vi "humidity_sensing_v_2.vi"() -> ()   [LabVIEW 2014]
doc: "This example shows how to configure a measurement and take a reading."
uses:
  <instrlib>/Keithley 24XX/Public/Data/Read (Single Point).vi
  <instrlib>/Keithley 24XX/Keithley 24XX.lvlib
panel:
  in  "current multiplier":dbl=1000000.0
  out "Resistance Data":string
  in  "Resistance Data":path=path "C:/Users/Administrator/Documents/humidity_sensing_setup/data/dumb/data_dumb_1.txt"
  out "Current Data":string
  in  "Current Data":path=path "C:/Users/Administrator/Documents/humidity_sensing_setup/data/dumb/data_dumb.txt"
  in  "stop":bool
  in  "Sampling rate (ms/pt)":i32=1000
  out "Current Data Graph":sgl(graph)=0.0001831192
  out "Resistance Data Graph":sgl(graph)=5460.51
  in  "loop num":dbl=10000000000.0
  in  "Stop Voltage/Current":dbl=1.0
  in  "Step":dbl
  in  "Source Mode  (0: Voltage)":u16(ring) items=["Voltage", "Current"]
  in  "Compliance  Level (0.1)":dbl=1.0
  in  "Start Voltage/Current":dbl=1.0
  in  "Enable Resistance Auto Range (T:Enable)":bool
  in  "Enable Current Auto Range (T:Enable)":bool=TRUE
  in  "Enable Voltage Auto Range (T:Enable)":bool
  in  "Resistance Manual Range (1.0)":dbl=1.0
  in  "Current Manual Range (1.0)":dbl=1.0
  in  "Voltage Manual Range (1.0)":dbl=1.0
  out "Resistance":sgl
  out "Current":sgl
  out "Voltage":sgl
  in  "Serial Configuration":T1={"Baud Rate"=9600, "Parity"=0, "Data Bits"=8, "Stop Bits"=10, "Flow Control"=0} {"Flow Control" items=["None", "XON/XOFF", "RTS/CTS", "XON/XOFF & RTS/CTS", "DTR/DSR", "XON/XOFF & DTR/DSR"]; "Stop Bits" items=["1.0"=10, "1.5"=15, "2.0"=20]; "Data Bits" items=["7"=7, "8"=8]; "Parity" items=["None", "Odd", "Even", "Mark", "Space"]; "Baud Rate" items=["300"=300, "600"=600, "1200"=1200, "2400"=2400, "4800"=4800, "9600"=9600, "19200"=19200]}
  in  "VISA resource name":refnum<visa-resource-name>="GPIB9::24::INSTR"
  # "NanoBEEs 2016-Humidity Chamber Setup v2.0"
  # "Source Settings"
  # "GPIB9::24::INSTR"
  # "Voltage Range Settings"
  # "Current Range Settings"
  # "This multiplies the current value\nwith the number that entered, in order\nto  graph lower current values."
  # "Resistance Range Settings"
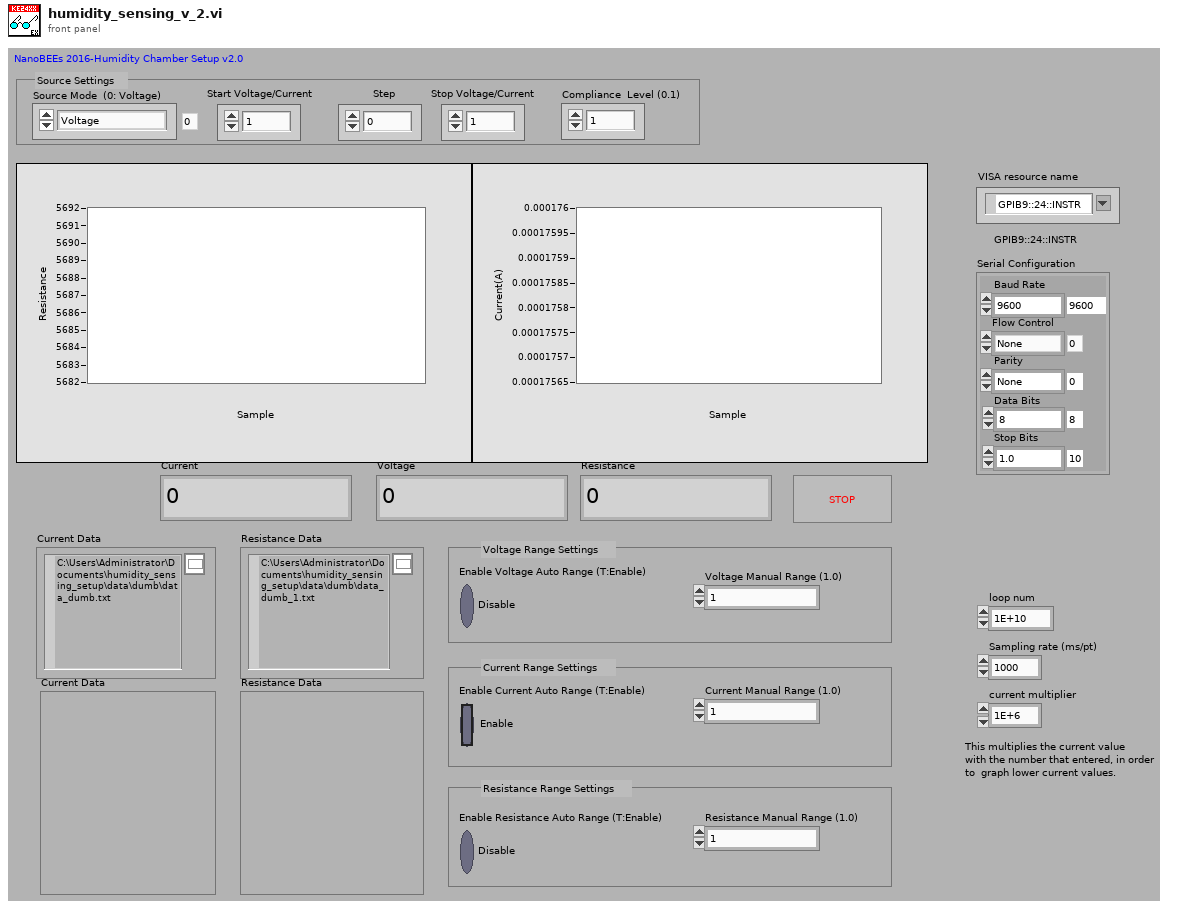
[diagram p1: front panel]
types:
  T1 = cluster{"Baud Rate":u32, "Parity":u16, "Data Bits":u16, "Stop Bits":u16, "Flow Control":u16}
  T2 = enum16{"open", "replace", "create", "open or create", "replace or create", "replace or create with confirmation"}
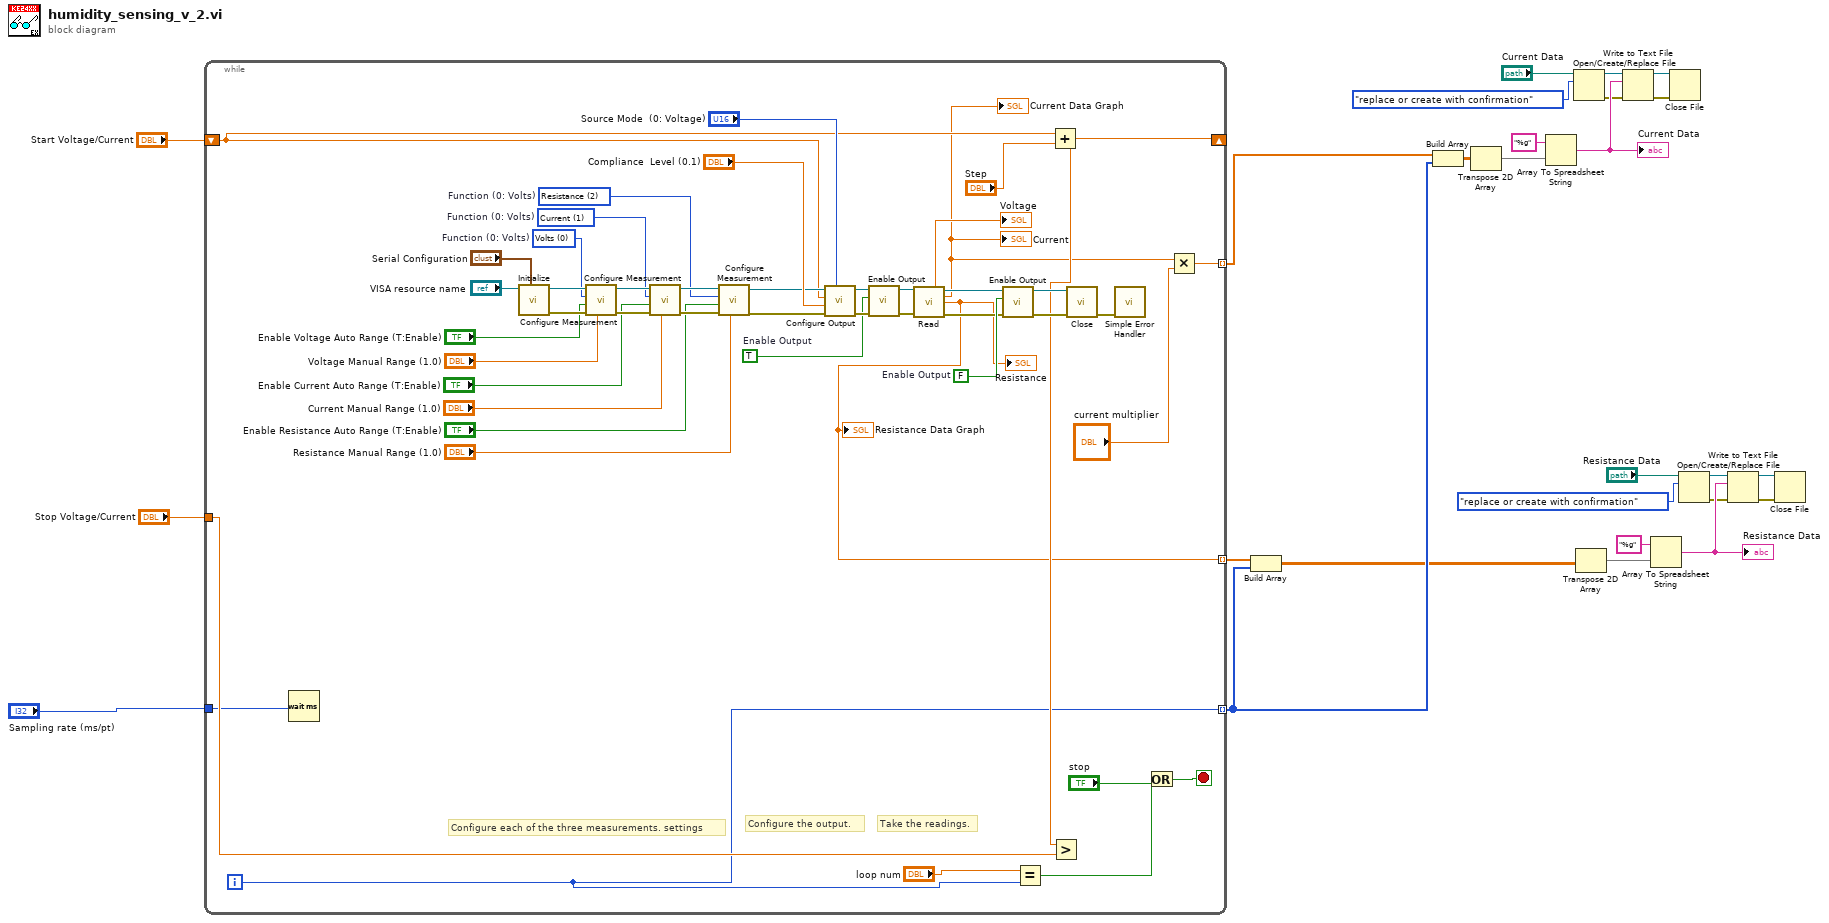
[diagram p0: block diagram]
diagram:
  n1 = while {
    shift-right: [w38] -> _
    shift-left: "Start Voltage/Current" -> [w41]
    tunnel: "Stop Voltage/Current" -> [w39]
    tunnel: "Sampling rate (ms/pt)" -> [w30]
    tunnel: [w34] -> w23 mode=indexing
    tunnel: [w31] -> w11 mode=indexing
    tunnel: [w29] -> w12 mode=indexing
    i -> [w31]
    stop <- w32 stop-if-true
    w45 = TRUE  # Enable Output
    w55 = FALSE  # Enable Output
    w62 = u16 2 items=["Volts", "Current", "Resistance"]  # Function (0: Volts)
    w63 = u16 1 items=["Volts", "Current", "Resistance"]  # Function (0: Volts)
    w64 = u16 0 items=["Volts", "Current", "Resistance"]  # Function (0: Volts)
    # "Take the readings."
    # "Configure the output."
    # "Configure each of the three measurements. settings"
    n2 = Wait (ms)(milliseconds to wait=w30) -> ()  [unwired: 1 out]
    n3 = call <instrlib>:"Initialize.vi"("Serial Configuration"="Serial Configuration", "VISA resource name"="VISA resource name") -> ("error out"=w69:errorcluster, "VISA resource name out"=w70:refnum<visa-resource-name>)  [unwired: 8 in]
    n4 = call <instrlib>:"Configure Measurement.vi"("Manual Range (1.0)"="Voltage Manual Range (1.0)", "error in (no error)"=w69, "Enable Auto Range (T:Enable)"="Enable Voltage Auto Range (T:Enable)", "Function (0: Volts)"=w64, "VISA resource name"=w70) -> ("error out"=w67:errorcluster, "VISA resource name out"=w68:refnum<visa-resource-name>)  [unwired: 5 in]
    n5 = call <instrlib>:"Configure Measurement.vi"("Manual Range (1.0)"="Current Manual Range (1.0)", "error in (no error)"=w67, "Enable Auto Range (T:Enable)"="Enable Current Auto Range (T:Enable)", "Function (0: Volts)"=w63, "VISA resource name"=w68) -> ("error out"=w66:errorcluster, "VISA resource name out"=w65:refnum<visa-resource-name>)  [unwired: 5 in]
    n6 = call <instrlib>:"Configure Measurement.vi"("Manual Range (1.0)"="Resistance Manual Range (1.0)", "error in (no error)"=w66, "Enable Auto Range (T:Enable)"="Enable Resistance Auto Range (T:Enable)", "Function (0: Volts)"=w62, "VISA resource name"=w65) -> ("error out"=w44:errorcluster, "VISA resource name out"=w43:refnum<visa-resource-name>)  [unwired: 5 in]
    n7 = call <instrlib>:"Configure Output.vi"("Source Mode  (0: Voltage)"="Source Mode  (0: Voltage)", "error in (no error)"=w44, "Compliance  Level (0.1)"="Compliance  Level (0.1)", "Output Level (0)"=w41, "VISA resource name"=w43) -> ("error out"=w46:errorcluster, "VISA resource name out"=w47:refnum<visa-resource-name>)  [unwired: 5 in]
    n8 = call <instrlib>:"Enable Output.vi"("error in (no error)"=w46, "Enable Output (T: Enable)"=w45, "VISA resource name"=w47) -> ("error out"=w49:errorcluster, "VISA resource name out"=w48:refnum<visa-resource-name>)  [unwired: 7 in]
    n9 = call-poly <instrlib>:"Read.vi"("VISA resource name"=w48, "error in (no error)"=w49) -> ("Voltage"=→"Voltage":sgl, "VISA resource name out"=w50:refnum<visa-resource-name>, "Current"=w28:sgl, "Resistance"=w34:sgl, "error out"=w51:errorcluster)  [unwired: 7 in, 2 out]
    "Current" <- w28
    "Resistance" <- w34
    "Resistance Data Graph" <- w34
    "Current Data Graph" <- w28
    n10 = call <instrlib>:"Enable Output.vi"("error in (no error)"=w51, "Enable Output (T: Enable)"=w55, "VISA resource name"=w50) -> ("error out"=w52:errorcluster, "VISA resource name out"=w53:refnum<visa-resource-name>)  [unwired: 7 in]
    n11 = Equal?(x="loop num", y=w31) -> (x = y?=w33:bool)
    n12 = Add(x=w41, y="Step") -> (x+y=w38:dbl)
    n13 = Greater?(x=w38, y=w39) -> ()  [unwired: 1 out]
    n14 = call <instrlib>:"Close.vi"("error in (no error)"=w52, "VISA resource name"=w53) -> ("error out"=w73:errorcluster)  [unwired: 9 in]
    n15 = call <vilib>:"Simple Error Handler.vi"("error in (no error)"=w73) -> ()  [unwired: 4 in, 5 out]
    n16 = Or(x=w33, y="stop") -> (x .or. y?=w32:bool)
    n17 = Multiply(x=w28, y="current multiplier") -> (x*y=w29:dbl)
  }
  n18 = Build Array(w23, w11) -> (w1:sgl[][])
  n19 = Build Array(w12, w11) -> (w19:dbl[][])
  n20 = Transpose 2D Array(2D array=w19) -> (transposed array=w21:dbl[][])
  n21 = Array To Spreadsheet String(array=w21, 3:"%g" ("format string")) -> (spreadsheet string=w22:string)  [unwired: 1 in]
  "Current Data" <- w22
  n22 = Open/Create/Replace File(file path (use dialog)="Current Data", operation (0:open)=T2."replace or create with confirmation") -> (refnum out=w18:refnum<file>, error out=w13:errorcluster)  [unwired: 4 in, 1 out]
  n23 = Transpose 2D Array(2D array=w1) -> (transposed array=w9:sgl[][])
  n24 = Write to Text File(file (use dialog)=w18, text=w22, error in=w13) -> (refnum out=w15:refnum<file>, error out=w14:errorcluster)  [unwired: 2 out]
  n25 = Array To Spreadsheet String(array=w9, 3:"%g" ("format string")) -> (spreadsheet string=w10:string)  [unwired: 1 in]
  "Resistance Data" <- w10
  n26 = Close File(refnum=w15, error in=w14) -> ()  [unwired: 2 out]
  n27 = Open/Create/Replace File(file path (use dialog)="Resistance Data", operation (0:open)=T2."replace or create with confirmation") -> (refnum out=w7:refnum<file>, error out=w2:errorcluster)  [unwired: 4 in, 1 out]
  n28 = Write to Text File(file (use dialog)=w7, text=w10, error in=w2) -> (refnum out=w4:refnum<file>, error out=w3:errorcluster)  [unwired: 2 out]
  n29 = Close File(refnum=w4, error in=w3) -> ()  [unwired: 2 out]
